vi "Write Coords.vi"(10 "Coordinates":T1, 11 "Handle Drag Over Msg in":refnum<class "Handle Drag Over Msg.lvclass">) -> (3 "Handle Drag Over Msg out":refnum<class "Handle Drag Over Msg.lvclass">)   [LabVIEW 2017, in "Handle Drag Over Msg.lvclass"]
uses:
  <vilib>/gpm_packages/@cs/Test-executive-builder/Source/Test Executive Builder View/Test Executive Builder View Messages/Handle Drag Over Msg/Handle Drag Over Msg.lvclass
  <vilib>/Utility/miscctls.llb/LVPoint32TypeDef.ctl
  <vilib>/gpm_packages/@cs/Test-executive-builder/Source/Test Executive Builder View/Test Executive Builder View Messages/Handle Drag Over Msg/Handle Drag Over Msg.lvclass/Handle Drag Over Msg.ctl
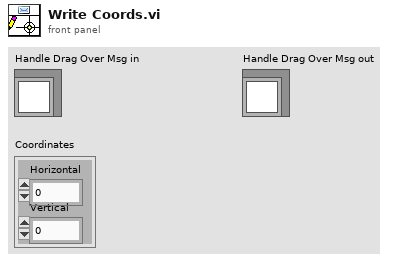
[diagram p1: front panel]
types:
  T1 = typedef "LVPoint32TypeDef.ctl" = cluster{"Horizontal":i32, "Vertical":i32}
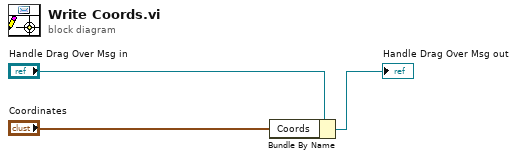
[diagram p0: block diagram]
diagram:
  n1 = Bundle By Name(cluster="Handle Drag Over Msg in", "Coords"="Coordinates") -> (→"Handle Drag Over Msg out":refnum<class "Handle Drag Over Msg.lvclass">)
